vi "接收数据量.vi"(0 "数值":u32) -> (1 "字符串":string, 2 "x*y":i32)   [LabVIEW 2016]
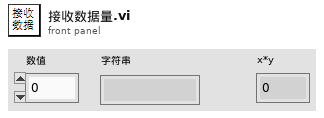
[diagram p1: front panel]
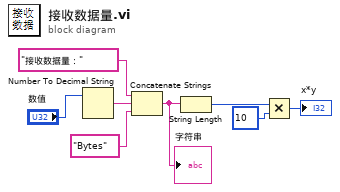
[diagram p0: block diagram]
diagram:
  n1 = Number To Decimal String(number="数值") -> (decimal integer string=w8:string)  [unwired: 1 in]
  n2 = Concatenate Strings("接收数据量：" ("字符串"), w8, "Bytes" ("字符串")) -> (w4:string)
  "字符串" <- w4
  n3 = String Length(string=w4) -> (length=w3:i32)
  n4 = Multiply(x=w3, y=10) -> (x*y=→"x*y":i32)
